vi "Init.vi"() -> (3 "TEMPLATE Msg Strategy out":refnum<class "TEMPLATE Msg Strategy.lvclass">)   [LabVIEW 2021, in "_Template.lvlib" / "Templates.lvlib" / "TEMPLATE Msg Strategy.lvlib" / "TEMPLATE Msg Strategy.lvclass"]
uses:
  TEMPLATE Msg Strategy.lvclass
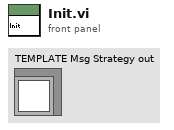
[diagram p1: front panel]
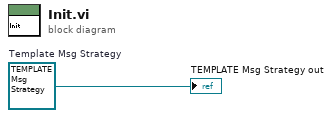
[diagram p0: block diagram]
diagram:
  w1 = refnum<class "TEMPLATE Msg Strategy.lvclass"> refnum  # Template Msg Strategy
  "TEMPLATE Msg Strategy out" <- w1
